vi "Set Pulse_Width.vi"(7 "Simulation":T2, 8 "error in":errorcluster, 9 "String":string, 10 "Args":string[](array[string]), 11 "Ophir Pulsar in":refnum<class "Ophir Pulsar.lvclass">) -> (0 "error out":errorcluster, 2 "new commands":string, 3 "Ophir Pulsar out":refnum<class "Ophir Pulsar.lvclass">)   [LabVIEW 2020, in "Ophir Pulsar.lvclass"]
uses:
  Ophir Pulsar.lvclass
  shared/OnOffTypeDef.ctl
  Controls/Pulse_Width.ctl
  Ophir Pulsar.lvclass/Ophir Pulsar.ctl
  shared/CompressAndUpdate(Poly)/CompressAndUpdate(Enum).vi
panel:
  in  "Pulse_Width":T1
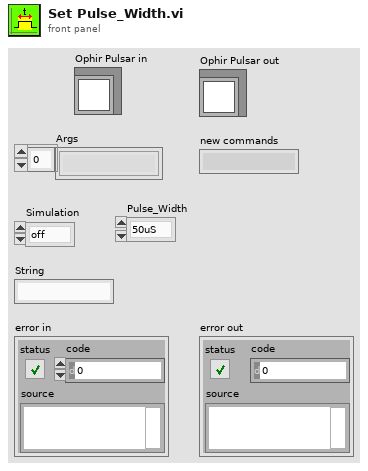
[diagram p1: front panel]
types:
  T1 = typedef "Ophir Pulsar.lvclass/Pulse_Width.ctl" = enum16{"50uS", "1.0mS"}
  T2 = typedef "OnOffTypeDef.ctl" = enum16{"off", "on"}
  T3 = cluster{"Channel0":T1, "Channel1":T1, "Channel2":T1, "Channel3":T1}
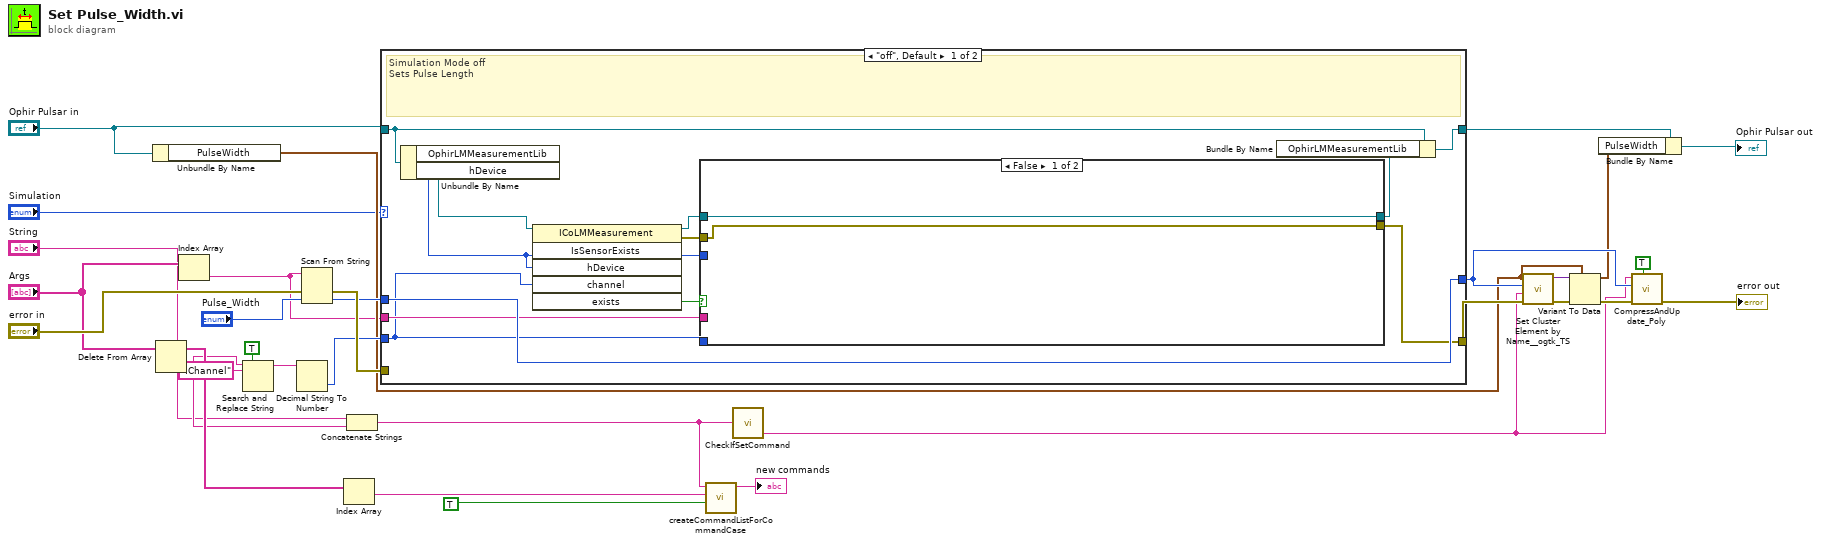
[diagram p0: block diagram]
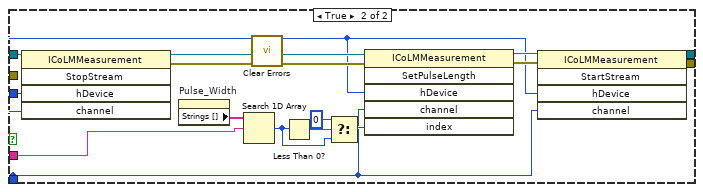
[diagram p2: hidden frame]
diagram:
  n1 = Unbundle By Name("Ophir Pulsar in") -> ("PulseWidth"=w14:T3)
  n2 = Delete From Array(array="Args") -> (deleted portion=w12:string, array with subset deleted=w18:string[])  [unwired: 2 in]
  n3 = Index Array(array="Args") -> (element=w1:string)  [unwired: 1 in]
  n4 = Search and Replace String(replace all?=TRUE ("replace all? (F)"), input string=w12, search string=".Channel") -> (result string=w16:string)  [unwired: 5 in, 3 out]
  n5 = Decimal String To Number(string=w16) -> (number=w30:i32)  [unwired: 2 in, 1 out]
  n6 = Scan From String(input string=w1, error in="error in", default 1="Pulse_Width") -> (error out=w31:errorcluster, output 1=w24:T1)  [unwired: 2 in, 2 out]
  n7 = Index Array(array=w18) -> (element=w19:string)  [unwired: 1 in]
  n8 = Concatenate Strings("String", w12) -> (w17:string)
  n9 = case shown="\"off\", Default" "Simulation" {
    tunnel: w24 -> [w41 w64]
    tunnel: [w41 w64] -> w26
    tunnel: w31 -> [_ w63]
    tunnel: [w40 w63] -> w27
    tunnel: "Ophir Pulsar in" -> [w43 w62]
    tunnel: [w42 w62] -> w21
    tunnel: w30 -> [w34 _]
    tunnel: w1 -> [w38 _]
    frame "off", Default {
      # "Simulation Mode off\nSets Pulse Length"
      n10 = Unbundle By Name(w43) -> ("OphirLMMeasurementLib"=w37:refnum<k7>, "hDevice"=w35:i32)
      n11 = invoke class="ICoLMMeasurement" method="IsSensorExists"(reference=w37, "hDevice"=w35, "channel"=w34) -> (reference out=w36:refnum<k7>, error out=w32:errorcluster, "exists"=w33:bool)  [unwired: 3 in, 3 out]
      n12 = case shown="False" w33 {
        tunnel: [w45 w57] -> w40
        tunnel: [w44 w56] -> w39
        tunnel: w38 -> [_ w50]
        tunnel: w36 -> [w44 w48]
        tunnel: w35 -> [_ w47]
        tunnel: w34 -> [_ w46]
        tunnel: w32 -> [w45 _]
        frame False {
        }
        frame True {
          n13 = invoke class="ICoLMMeasurement" method="StopStream"(reference=w48, "hDevice"=w47, "channel"=w46) -> (reference out=w60:refnum<k7>, error out=w61:errorcluster)  [unwired: 2 in, 3 out]
          n14 = property on="Pulse_Width" class="Enum (strict)"() -> ("Strings []"=w55:string[])  [unwired: 2 in, 2 out]
          n15 = Search 1D Array(1D array=w55, element=w50) -> (index of element=w52:i32)  [unwired: 1 in]
          n16 = call <vilib>:"Clear Errors.vi"("error in (no error)"=w61) -> ("error out"=w49:errorcluster)  [unwired: 5 in, 1 out]
          n17 = Less Than 0?(x=w52) -> (x < 0?=w54:bool)
          n18 = Select(t=0, s=w54, f=w52) -> (s? t:f=w51:i32)
          n19 = invoke class="ICoLMMeasurement" method="SetPulseLength"(reference=w60, error in=w49, "hDevice"=w47, "channel"=w46, "index"=w51) -> (reference out=w59:refnum<k7>, error out=w58:errorcluster)  [unwired: 1 in, 4 out]
          n20 = invoke class="ICoLMMeasurement" method="StartStream"(reference=w59, error in=w58, "hDevice"=w47, "channel"=w46) -> (reference out=w56:refnum<k7>, error out=w57:errorcluster)  [unwired: 1 in, 3 out]
        }
      }
      n21 = Bundle By Name(cluster=w43, "OphirLMMeasurementLib"=w39) -> (w42:refnum<class "Ophir Pulsar.lvclass">)
    }
    frame "on" {
      # "Simulation Mode on"
    }
  }
  n22 = call "createCommandListForCommandCase.vi"("immediate Check (only once)"=TRUE, "setvalue"=w19, "command"=w17) -> ("new commands"=→"new commands":string)  [unwired: 8 in]
  n23 = call "CheckIfSetCommand.vi"("Command"=w17) -> ("variable"=w11:string)  [unwired: 2 out]
  n24 = call "Set Cluster Element by Name__ogtk_TS.vi"("error in (no error)"=w27, "Element Name (\"\": New Element Data Name)"=w11, "New Element Value"=w26, "Cluster"=w14) -> ("error out"=w28:errorcluster, "VCluster out"=w15:variant)  [unwired: 5 in, 1 out]
  n25 = Variant To Data(error in=w28, type=w14, Variant=w15) -> (data=w13:T3, error out=w29:errorcluster)
  n26 = Bundle By Name(cluster=w21, "PulseWidth"=w13) -> (→"Ophir Pulsar out":refnum<class "Ophir Pulsar.lvclass">)
  n27 = call-poly "CompressAndUpdate_Poly.vi"("force CVT update (false)"=TRUE, "error in"=w29, "enum variant"=w26, "command or variable name"=w11) -> ("error out"=→"error out":errorcluster)  [unwired: 7 in]
